vi "RunPump.vi"(8 "error in (no error)":errorcluster, 11 "VISA Refnum in":refnum<visa-resource-name>) -> (0 "error out":errorcluster, 3 "VISA Refnum out":refnum<visa-resource-name>)   [LabVIEW 2020]
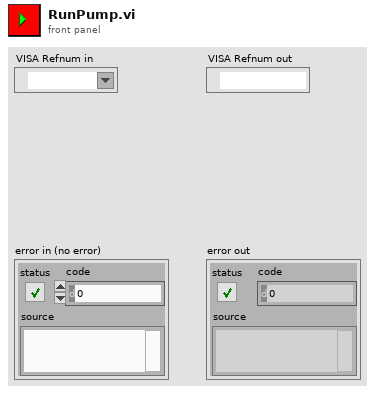
[diagram p1: front panel]
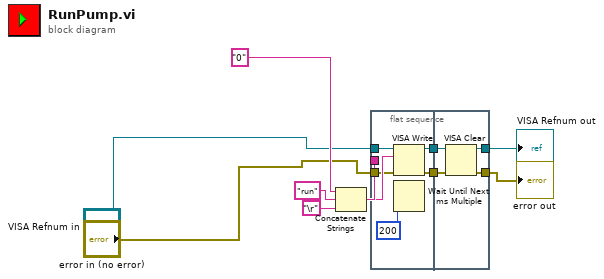
[diagram p0: block diagram]
diagram:
  n1 = Concatenate Strings("0" ("string"), "run" ("string"), "\r") -> (w3:string)
  n2 = flat-sequence {
    tunnel: w3 -> [w16]
    tunnel: "VISA Refnum in" -> [w15]
    tunnel: "error in (no error)" -> [w14]
    tunnel: [w13] -> w10
    tunnel: [w12] -> w9
    tunnel: w10 -> [w20]
    tunnel: w9 -> [w19]
    tunnel: [w18] -> w7
    tunnel: [w17] -> w8
    frame #0 {
      n3 = VISA Write(VISA resource name=w15, write buffer=w16, error in (no error)=w14) -> (VISA resource name out=w13:refnum<visa-resource-name>, error out=w12:errorcluster)  [unwired: 1 out]
      n4 = Wait Until Next ms Multiple(millisecond multiple=u32 200) -> ()  [unwired: 1 out]
    }
    frame #1 {
      n5 = VISA Clear(VISA resource name=w20, error in (no error)=w19) -> (VISA resource name out=w18:refnum<visa-resource-name>, error out=w17:errorcluster)
    }
  }
  "error out" <- w8
  "VISA Refnum out" <- w7
